vi "Start motor.vi"(8 "error in (no error)":errorcluster, 11 "VISA resource name":refnum<visa-resource-name>) -> (0 "error out":errorcluster, 3 "VISA resource name out":refnum<visa-resource-name>)   [LabVIEW 2018]
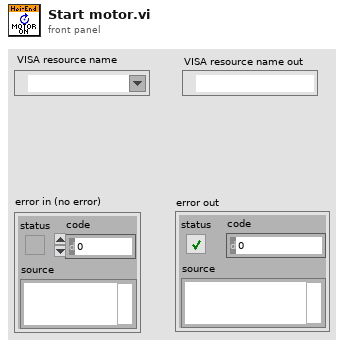
[diagram p1: front panel]
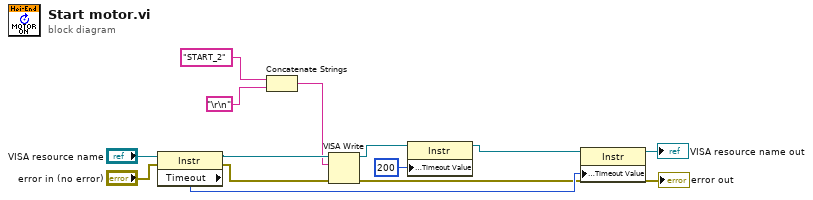
[diagram p0: block diagram]
diagram:
  n1 = property class="Instr"(reference="VISA resource name", error in="error in (no error)") -> (reference out=w10:refnum<visa-resource-name>, error out=w9:errorcluster, "Timeout"=w8:u32)
  n2 = Concatenate Strings("START_2" ("format string"), "\r\n") -> (w6:string)
  n3 = VISA Write(VISA resource name=w10, write buffer=w6, error in (no error)=w9) -> (VISA resource name out=w2:refnum<visa-resource-name>, error out=→"error out":errorcluster)  [unwired: 1 out]
  n4 = property class="Instr"(reference=w2, "General Settings:Timeout Value"=u32 200) -> (reference out=w1:refnum<visa-resource-name>)  [unwired: 1 in, 1 out]
  n5 = property class="Instr"(reference=w1, "General Settings:Timeout Value"=w8) -> (reference out=→"VISA resource name out":refnum<visa-resource-name>)  [unwired: 1 in, 1 out]
